vi "Inspect row from both ends.vi"(10 "Trees in":T1[](array[typedef])) -> (2 "Trees out":T1[](array[typedef]))   [LabVIEW 2020]
uses:
  tree--cluster.ctl
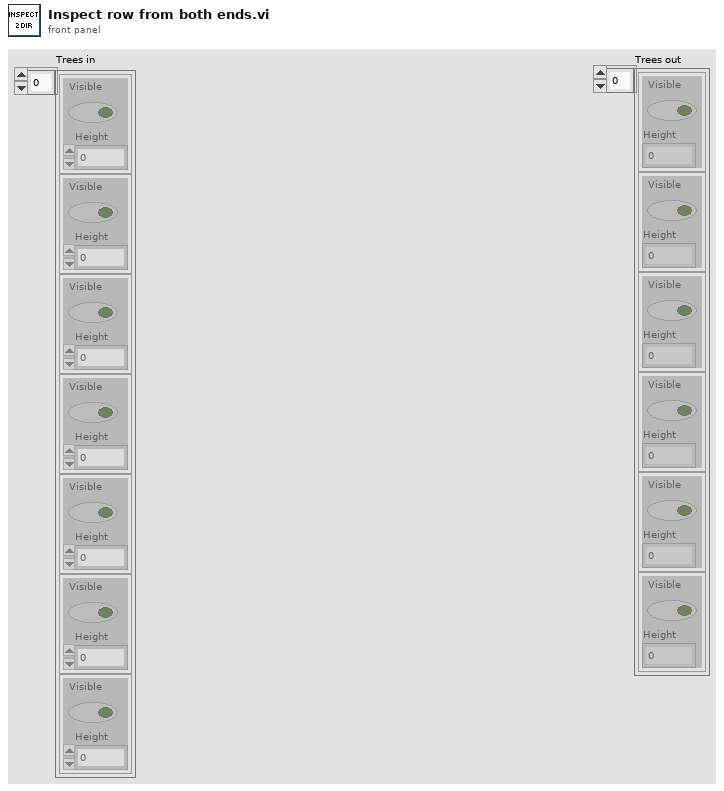
[diagram p1: front panel]
types:
  T1 = typedef "tree--cluster.ctl" = cluster{"Visible":bool, "Height":i32}
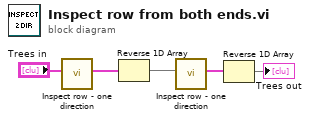
[diagram p0: block diagram]
diagram:
  n1 = call "Inspect row - one direction.vi"("Trees in"="Trees in") -> ("Trees out"=w4:T1[])  [unwired: 10 in]
  n2 = Reverse 1D Array(array=w4) -> (reversed array=w3:T1[])
  n3 = call "Inspect row - one direction.vi"("Trees in"=w3) -> ("Trees out"=w2:T1[])  [unwired: 10 in]
  n4 = Reverse 1D Array(array=w2) -> (reversed array=→"Trees out":T1[])
